vi "Read As Stream_Start.vi"(8 "error in (no error)":errorcluster, 10 "DestinationStream":refnum<k24>, 11 "HttpContent in":refnum<class "HttpContent.lvclass">) -> (0 "error out":errorcluster, 3 "HttpContent out":refnum<class "HttpContent.lvclass">)   [LabVIEW 2018, in "LabVIEWHTTPClient_NET.lvlib" / "HttpContent.lvclass"]
uses:
  HttpContent.lvclass
  HttpContent.lvclass/HttpContent.ctl
  System.Net.Http
  Accessors/Read NET_HttpContent.vi
  Accessors/Read timeout_ms.vi
  Accessors/Write NET_StreamTask.vi
  Accessors/Write NET_StreamCancellationSource.vi
  Accessors/Write NET_SourceStream.vi
  Accessors/Write NET_DestinationStream.vi
  LabVIEWHTTPClient_NET/LabVIEWHTTPClient_NET.lvclass
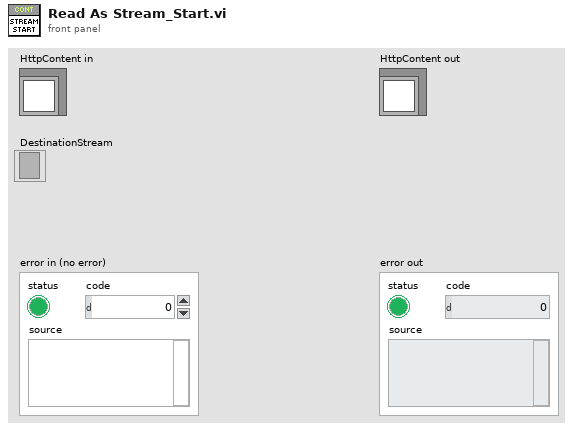
[diagram p1: front panel]
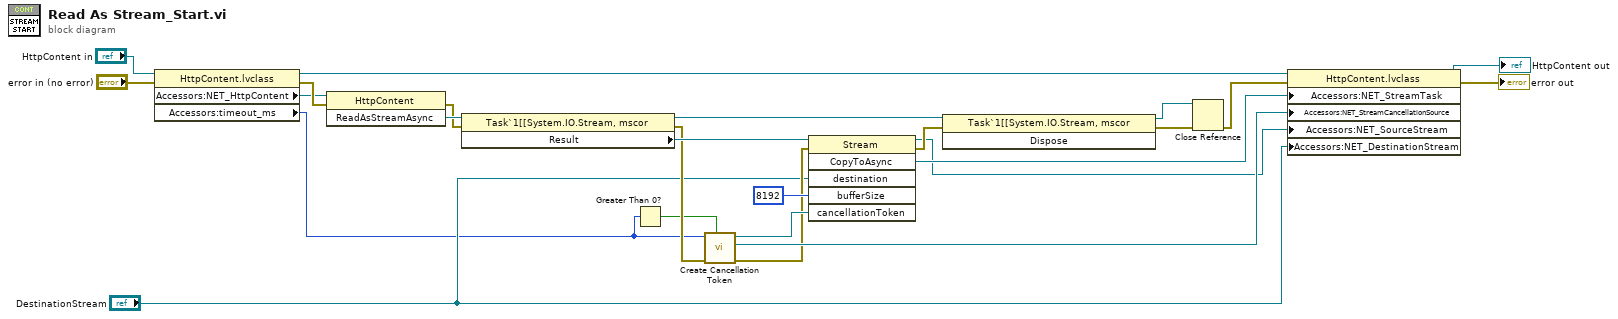
[diagram p0: block diagram]
diagram:
  n1 = property class="HttpContent.lvclass"(reference="HttpContent in", error in="error in (no error)") -> (reference out=w12:refnum<class "HttpContent.lvclass">, error out=w25:errorcluster, "Accessors:NET_HttpContent"=w24:refnum<k24>, "Accessors:timeout_ms"=w2:i32)
  n2 = invoke class="HttpContent" method="ReadAsStreamAsync"(reference=w24, error in=w25) -> (error out=w17:errorcluster, "ReadAsStreamAsync"=w22:refnum<k24>)  [unwired: 1 in, 1 out]
  n3 = property class="Task`1[[System.IO.Stream, mscor"(reference=w22, error in=w17) -> (reference out=w20:refnum<k24>, error out=w5:errorcluster, "Result"=w21:refnum<k24>)
  n4 = Greater Than 0?(x=w2) -> (x > 0?=w1:bool)
  n5 = call "Create Cancellation Token.vi"("IncludeTimeout (T)"=w1, "error in (no error)"=w5, "Timeout_ms (10000)"=w2) -> ("error out"=w4:errorcluster, "NET_CancellationSource"=w9:refnum<k24>, "NET_CancellationToken"=w10:refnum<k24>)  [unwired: 6 in]
  n6 = invoke class="Stream" method="CopyToAsync"(reference=w21, error in=w4, "destination"="DestinationStream", "bufferSize"=8192, "cancellationToken"=w10) -> (reference out=w7:refnum<k24>, error out=w16:errorcluster, "CopyToAsync"=w8:refnum<k24>)  [unwired: 1 in, 3 out]
  n7 = invoke class="Task`1[[System.IO.Stream, mscor" method="Dispose"(reference=w20, error in=w16) -> (reference out=w18:refnum<k24>, error out=w19:errorcluster)  [unwired: 1 in, 1 out]
  n8 = Close Reference(reference=w18, error in (no error)=w19) -> (error out=w14:errorcluster)
  n9 = property class="HttpContent.lvclass"(reference=w12, error in=w14, "Accessors:NET_StreamTask"=w8, "Accessors:NET_StreamCancellationSource"=w9, "Accessors:NET_SourceStream"=w7, "Accessors:NET_DestinationStream"="DestinationStream") -> (reference out=→"HttpContent out":refnum<class "HttpContent.lvclass">, error out=→"error out":errorcluster)
